vi "MARATHON_CAPACITY TEST.vi"() -> ()   [LabVIEW 2017]
uses:
  <userlib>/LV-Link3/PolySubVIs/DtOLTimingSetInput.vi
  <userlib>/LV-Link3/PolySubVIs/DtOLReadMultiple2D.vi
panel:
  in  "Limit Cell Voltage":dbl[](array[numeric]) format="%_4g"
  out "x+y 2":dbl[](array[numeric])
  out "x+y":dbl[](array[knob]) scale=0.0..32.0
  out "Time 20":dbl format="%<%H:%M:%S>t"
  out "Time 19":dbl format="%<%H:%M:%S>t"
  out "Time 18":dbl format="%<%H:%M:%S>t"
  out "Time 17":dbl format="%<%H:%M:%S>t"
  out "Time 16":dbl format="%<%H:%M:%S>t"
  out "Time 15":dbl format="%<%H:%M:%S>t"
  out "Time 14":dbl format="%<%H:%M:%S>t"
  out "Time 13":dbl format="%<%H:%M:%S>t"
  out "Time 12":dbl format="%<%H:%M:%S>t"
  out "Time 11":dbl format="%<%H:%M:%S>t"
  out "Time 10":dbl format="%<%H:%M:%S>t"
  out "Time 9":dbl format="%<%H:%M:%S>t"
  out "Time 8":dbl format="%<%H:%M:%S>t"
  out "Time 7":dbl format="%<%H:%M:%S>t"
  out "Time 6":dbl format="%<%H:%M:%S>t"
  out "Time 5":dbl format="%<%H:%M:%S>t"
  out "Time 4":dbl format="%<%H:%M:%S>t"
  out "Time 3":dbl format="%<%H:%M:%S>t"
  out "Time 2":dbl format="%<%H:%M:%S>t"
  out "Time 1":dbl format="%<%H:%M:%S>t"
  out "CELL #19":bool[](array[boolean])
  out "CELL #20":bool[](array[boolean])
  out "CELL #18":bool[](array[boolean])
  out "CELL #17":bool[](array[boolean])
  out "CELL #16":bool[](array[boolean])
  out "CELL #15":bool[](array[boolean])
  out "CELL #14":bool[](array[boolean])
  out "CELL #13":bool[](array[boolean])
  out "CELL #12":bool[](array[boolean])
  out "CELL #11":bool[](array[boolean])
  out "CELL #10":bool[](array[boolean])
  out "CELL #9":bool[](array[boolean])
  out "CELL #8":bool[](array[boolean])
  out "CELL #7":bool[](array[boolean])
  out "CELL #6":bool[](array[boolean])
  out "CELL #5":bool[](array[boolean])
  out "CELL #4":bool[](array[boolean])
  out "CELL #3":bool[](array[boolean])
  out "CELL #2":bool[](array[boolean])
  out "CELL #1":bool[](array[boolean])
  out "VOLT # 20":dbl[](array[numeric])
  out "VOLT # 19":dbl[](array[numeric])
  out "VOLT # 18":dbl[](array[numeric])
  out "VOLT # 17":dbl[](array[numeric])
  out "VOLT # 16":dbl[](array[numeric])
  out "VOLT # 15":dbl[](array[numeric])
  out "VOLT # 14":dbl[](array[numeric])
  out "VOLT # 13":dbl[](array[numeric])
  out "VOLT # 12":dbl[](array[numeric])
  out "VOLT # 11":dbl[](array[numeric])
  out "VOLT # 10":dbl[](array[numeric])
  out "VOLT # 9":dbl[](array[numeric])
  out "VOLT # 8":dbl[](array[numeric])
  out "VOLT # 7":dbl[](array[numeric])
  out "VOLT # 6":dbl[](array[numeric])
  out "VOLT # 5":dbl[](array[numeric])
  out "VOLT # 4":dbl[](array[numeric])
  out "VOLT # 3":dbl[](array[numeric])
  out "VOLT # 2":dbl[](array[numeric])
  out "VOLT # 1":dbl[](array[numeric])
  in  "POWER":bool caption="START"
  in  "stop":bool
  # "FLUKE"
  # "179 Multimeter"
  # "28.56789 VOLTS"
  # "SuperMasterCharger"
  # "Time"
  # "Current"
  # "Hold"
  # "Range"
  # "ON"
  # "04:56"
  # "000.7"
  # "R"
  # "20 CELLS"
  # "mV"
  # "Voltage"
  # "D"
  # "V--"
  # "STATUS"
  # "CAP TEST"
  # "A--"
  # "OFF"
  # "Jfm"
  # "1"
  # "Run"
  # "2"
  # "3"
  # "M"
  # "T"
  # "4"
  # "6"
  # "B"
  # "ST"
  # "5"
  # "CU"
  # "SAFT"
  # "8"
  # "OPT"
  # "V"
  # "RST"
  # "7"
  # "9"
  # "Vie"
  # "FN"
  # "ENT"
  # "0"
  # "C"
  # "P"
  # "POWER"
  # "Harness"
  # "WATER"
  # "ACID"
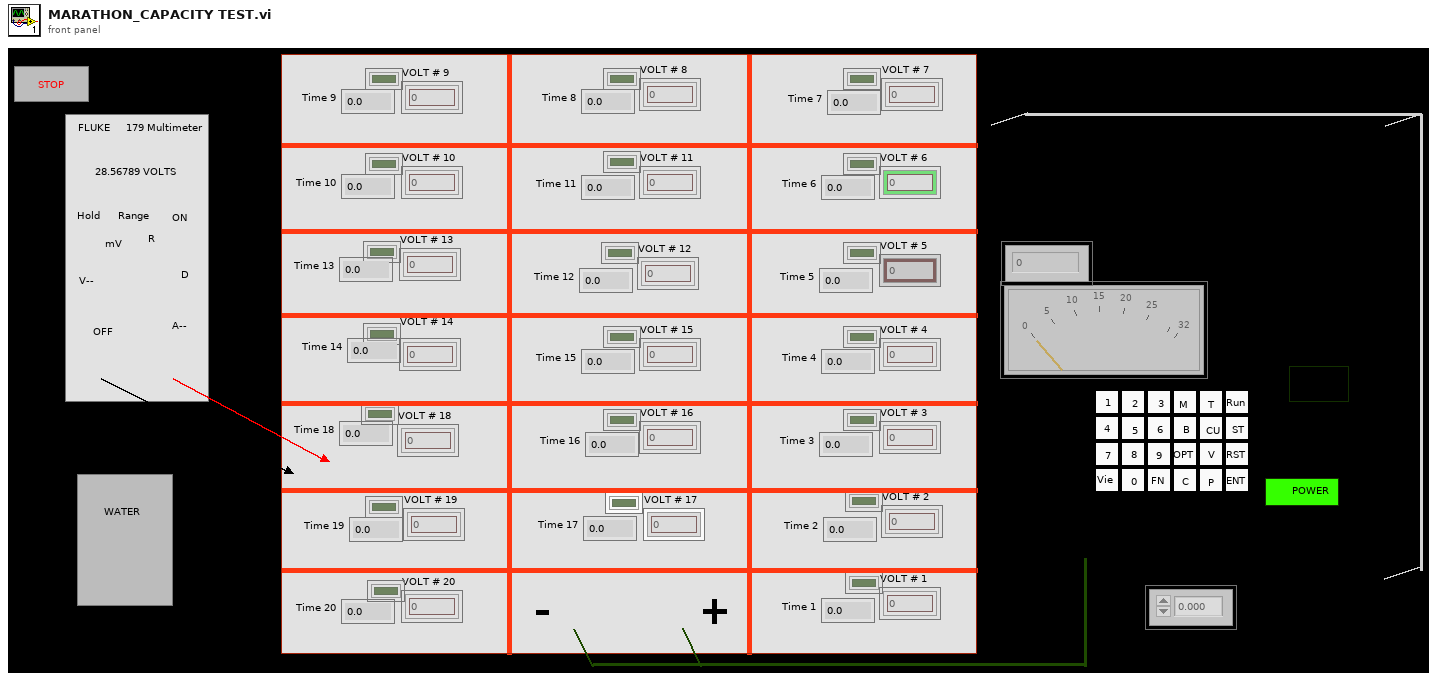
[diagram p1: front panel]
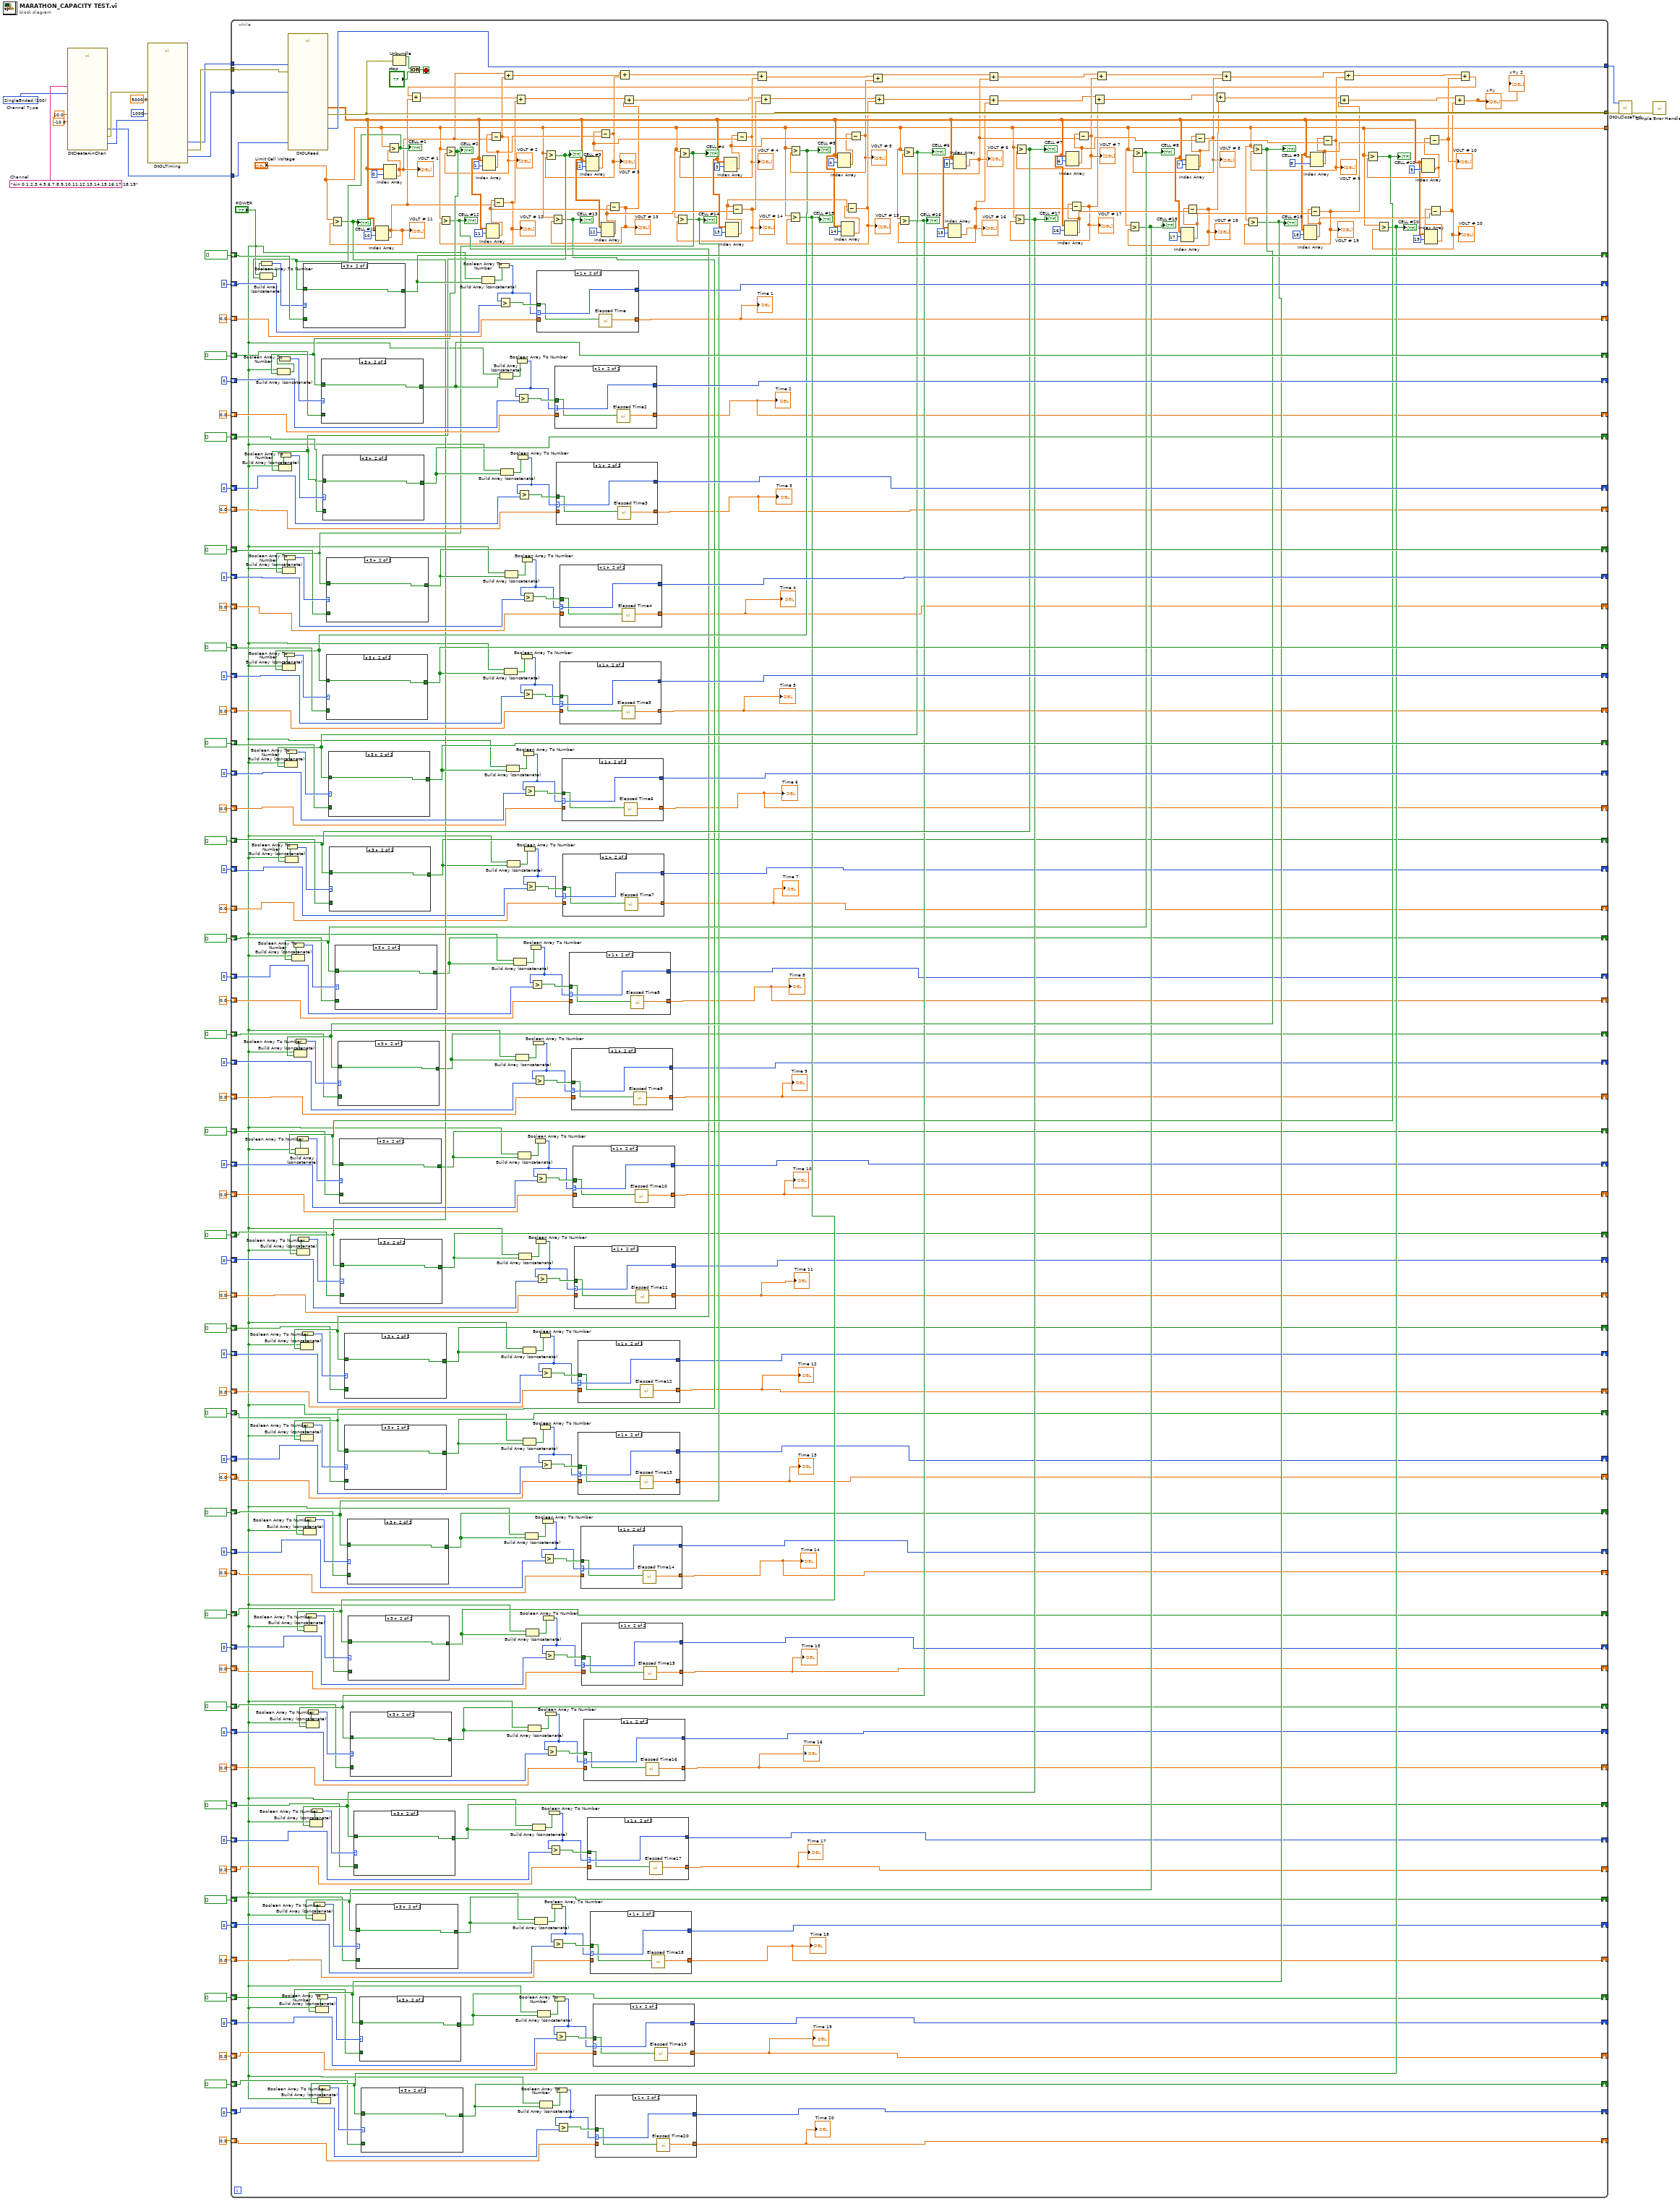
[diagram p0: block diagram]
diagram:
  w75 = 100 items=["Differential"=101, "SingleEnded"=100]  # Channel Type
  w72 = "Ain 0,1,2,3,4,5,6,7,8,9,10,11,12,13,14,15,16,17,18,19"  # Channel
  n1 = call <userlib>:"DtCreateAinChan.vi"("Channel Type"=w75, "Range Min"=-10.0, "Range Max"=10.0, "Channel"=w72) -> ("Task out"=w62:i32, "Actual Number of Channels"=w61:u32, "error out"=w71:errorcluster)  [unwired: 9 in]
  n2 = call-poly <userlib>:"DtOLTiming.vi"("Samples Per Channel"=u32 1000, "error in (no error)"=w71, "Sample Freq (Hz)"=5000.0, "Task in"=w62) -> ("error out"=w68:errorcluster, "Buffer Size"=w67:u32, "Task out"=w66:i32)  [unwired: 4 in, 1 out]
  n3 = while {
    tunnel: w68 -> [w402]
    tunnel: w67 -> [w400]
    tunnel: w66 -> [w401]
    tunnel: [w397] -> w65
    tunnel: [w398] -> w64
    tunnel: w61 -> [w396]
    shift-right: [w255] -> _
    shift-left: bool[] [] -> [w354]
    shift-right: [w214] -> _
    shift-left: u32 0 -> [w353]
    shift-right: [w99] -> _
    shift-left: 0.0 ("Elapsed Time (s)") -> [w352]
    shift-right: [w254] -> _
    shift-left: bool[] [] -> [w253]
    shift-right: [w251] -> _
    shift-left: u32 0 -> [w250]
    shift-right: [w94] -> _
    shift-left: 0.0 ("Elapsed Time (s)") -> [w249]
    shift-right: [w248] -> _
    shift-left: bool[] [] -> [w247]
    shift-right: [w246] -> _
    shift-left: u32 0 -> [w245]
    shift-right: [w93] -> _
    shift-left: 0.0 ("Elapsed Time (s)") -> [w244]
    shift-right: [w243] -> _
    shift-left: bool[] [] -> [w242]
    shift-right: [w241] -> _
    shift-left: u32 0 -> [w240]
    shift-right: [w92] -> _
    shift-left: 0.0 ("Elapsed Time (s)") -> [w239]
    shift-right: [w238] -> _
    shift-left: bool[] [] -> [w236]
    shift-right: [w237] -> _
    shift-left: u32 0 -> [w235]
    shift-right: [w91] -> _
    shift-left: 0.0 ("Elapsed Time (s)") -> [w234]
    shift-right: [w233] -> _
    shift-left: bool[] [] -> [w232]
    shift-right: [w231] -> _
    shift-left: u32 0 -> [w230]
    shift-right: [w90] -> _
    shift-left: 0.0 ("Elapsed Time (s)") -> [w229]
    shift-right: [w206] -> _
    shift-left: bool[] [] -> [w205]
    shift-right: [w204] -> _
    shift-left: u32 0 -> [w203]
    shift-right: [w89] -> _
    shift-left: 0.0 ("Elapsed Time (s)") -> [w202]
    shift-right: [w201] -> _
    shift-left: bool[] [] -> [w175]
    shift-right: [w200] -> _
    shift-left: u32 0 -> [w174]
    shift-right: [w88] -> _
    shift-left: 0.0 ("Elapsed Time (s)") -> [w173]
    shift-right: [w199] -> _
    shift-left: bool[] [] -> [w172]
    shift-right: [w198] -> _
    shift-left: u32 0 -> [w171]
    shift-right: [w87] -> _
    shift-left: 0.0 ("Elapsed Time (s)") -> [w170]
    shift-right: [w197] -> _
    shift-left: bool[] [] -> [w169]
    shift-right: [w196] -> _
    shift-left: u32 0 -> [w168]
    shift-right: [w86] -> _
    shift-left: 0.0 ("Elapsed Time (s)") -> [w167]
    shift-right: [w195] -> _
    shift-left: bool[] [] -> [w166]
    shift-right: [w194] -> _
    shift-left: u32 0 -> [w165]
    shift-right: [w85] -> _
    shift-left: 0.0 ("Elapsed Time (s)") -> [w164]
    shift-right: [w193] -> _
    shift-left: bool[] [] -> [w163]
    shift-right: [w192] -> _
    shift-left: u32 0 -> [w162]
    shift-right: [w84] -> _
    shift-left: 0.0 ("Elapsed Time (s)") -> [w161]
    shift-right: [w191] -> _
    shift-left: bool[] [] -> [w160]
    shift-right: [w190] -> _
    shift-left: u32 0 -> [w159]
    shift-right: [w83] -> _
    shift-left: 0.0 ("Elapsed Time (s)") -> [w158]
    shift-right: [w189] -> _
    shift-left: bool[] [] -> [w157]
    shift-right: [w188] -> _
    shift-left: u32 0 -> [w156]
    shift-right: [w82] -> _
    shift-left: 0.0 ("Elapsed Time (s)") -> [w155]
    shift-right: [w187] -> _
    shift-left: bool[] [] -> [w154]
    shift-right: [w186] -> _
    shift-left: u32 0 -> [w153]
    shift-right: [w81] -> _
    shift-left: 0.0 ("Elapsed Time (s)") -> [w152]
    shift-right: [w185] -> _
    shift-left: bool[] [] -> [w151]
    shift-right: [w184] -> _
    shift-left: u32 0 -> [w150]
    shift-right: [w80] -> _
    shift-left: 0.0 ("Elapsed Time (s)") -> [w149]
    shift-right: [w183] -> _
    shift-left: bool[] [] -> [w148]
    shift-right: [w182] -> _
    shift-left: u32 0 -> [w147]
    shift-right: [w79] -> _
    shift-left: 0.0 ("Elapsed Time (s)") -> [w146]
    shift-right: [w181] -> _
    shift-left: bool[] [] -> [w145]
    shift-right: [w180] -> _
    shift-left: u32 0 -> [w144]
    shift-right: [w78] -> _
    shift-left: 0.0 ("Elapsed Time (s)") -> [w143]
    shift-right: [w179] -> _
    shift-left: bool[] [] -> [w142]
    shift-right: [w178] -> _
    shift-left: u32 0 -> [w141]
    shift-right: [w77] -> _
    shift-left: 0.0 ("Elapsed Time (s)") -> [w140]
    shift-right: [w177] -> _
    shift-left: bool[] [] -> [w139]
    shift-right: [w176] -> _
    shift-left: u32 0 -> [w138]
    shift-right: [w76] -> _
    shift-left: 0.0 ("Elapsed Time (s)") -> [w137]
    tunnel: ["Limit Cell Voltage"] -> _
    stop <- w374 stop-if-true
    n4 = call-poly <userlib>:"DtOLRead.vi"("Number Chan to Read"=w396, "Buffer size"=w400, "error in (no error)"=w402, "Task in"=w401) -> ("error out"=w397:errorcluster, "2D Data out"=w373:dbl[][], "Task out"=w398:i32)  [unwired: 3 in, 2 out]
    n5 = Index Array(array=w373, index (row)=10) -> (element=w97:dbl[])  [unwired: 1 in]
    "VOLT # 11" <- w97
    n6 = Greater?(x="Limit Cell Voltage", y=w97) -> (0:w217:bool[])
    "CELL #11" <- w217
    n7 = Build Array (concatenate)("POWER", w217) -> (w302:bool[])
    n8 = Boolean Array To Number(Boolean array=w302) -> (number=w301:u32)
    n9 = case shown="3" w301 {
      tunnel: w217 -> [_ w472]
      tunnel: [w471 w472] -> w195
      tunnel: w166 -> [w471 _]
      frame 0, Default {
      }
      frame 3 {
      }
    }
    n10 = Index Array(array=w373, index (row)=0) -> (element=w135:dbl[])  [unwired: 1 in]
    "VOLT # 1" <- w135
    n11 = Greater?(x="Limit Cell Voltage", y=w135) -> (0:w228:bool[])
    "CELL #1" <- w228
    n12 = Build Array (concatenate)("POWER", w228) -> (w351:bool[])
    n13 = Boolean Array To Number(Boolean array=w351) -> (number=w350:u32)
    n14 = case shown="3" w350 {
      tunnel: w228 -> [_ w542]
      tunnel: [w541 w542] -> w255
      tunnel: w354 -> [w541 _]
      frame 0, Default {
      }
      frame 3 {
      }
    }
    n15 = Unbundle "Unbundle"(w397) -> ("status"=w399:bool)  [unwired: 2 out]
    n16 = Or(x=w399, y="stop") -> (x .or. y?=w374:bool)
    n17 = Build Array (concatenate)("POWER", w255) -> (w356:bool[])
    n18 = Index Array(array=w373, index (row)=1) -> (element=w372:dbl[])  [unwired: 1 in]
    n19 = Index Array(array=w373, index (row)=11) -> (element=w364:dbl[])  [unwired: 1 in]
    n20 = Subtract(x=w372, y=w135) -> (x-y=w134:dbl[])
    "VOLT # 2" <- w134
    n21 = Greater?(x="Limit Cell Voltage", y=w134) -> (0:w227:bool[])
    "CELL #2" <- w227
    n22 = Build Array (concatenate)("POWER", w227) -> (w252:bool[])
    n23 = Boolean Array To Number(Boolean array=w252) -> (number=w346:u32)
    n24 = case shown="3" w346 {
      tunnel: w227 -> [_ w535]
      tunnel: [w534 w535] -> w254
      tunnel: w253 -> [w534 _]
      frame 0, Default {
      }
      frame 3 {
      }
    }
    n25 = Subtract(x=w364, y=w97) -> (x-y=w116:dbl[])
    "VOLT # 12" <- w116
    n26 = Greater?(x="Limit Cell Voltage", y=w116) -> (0:w216:bool[])
    "CELL #12" <- w216
    n27 = Build Array (concatenate)("POWER", w216) -> (w297:bool[])
    n28 = Boolean Array To Number(Boolean array=w297) -> (number=w296:u32)
    n29 = case shown="3" w296 {
      tunnel: w216 -> [_ w465]
      tunnel: [w464 w465] -> w193
      tunnel: w163 -> [w464 _]
      frame 0, Default {
      }
      frame 3 {
      }
    }
    n30 = Boolean Array To Number(Boolean array=w356) -> (number=w355:u32)
    n31 = Greater?(x=w355, y=w353) -> (0:w357:bool)
    n32 = Build Array (concatenate)("POWER", w254) -> (w348:bool[])
    n33 = Add(x=w135, y=w134) -> (x+y=w133:dbl[])
    n34 = Boolean Array To Number(Boolean array=w348) -> (number=w347:u32)
    n35 = Greater?(x=w347, y=w250) -> (0:w349:bool)
    n36 = Build Array (concatenate)("POWER", w195) -> (w304:bool[])
    n37 = Build Array (concatenate)("POWER", w193) -> (w299:bool[])
    n38 = Boolean Array To Number(Boolean array=w304) -> (number=w303:u32)
    n39 = Greater?(x=w303, y=w165) -> (0:w305:bool)
    n40 = case shown="1" w355 {
      selector: w355 -> [w537 w539]
      tunnel: [w536 w540] -> w99
      tunnel: w352 -> [w536 _]
      tunnel: [w537 w539] -> w214
      tunnel: w357 -> [_ w538]
      frame 0, Default {
      }
      frame 1 {
        n41 = call "Elapsed Time"("Reset"=w538) -> ("Elapsed Time (s)"=w540:dbl)  [unwired: 11 in, 7 out]
      }
    }
    "Time 1" <- w99
    n42 = Boolean Array To Number(Boolean array=w299) -> (number=w298:u32)
    n43 = Greater?(x=w298, y=w162) -> (0:w300:bool)
    n44 = case shown="1" w347 {
      selector: w347 -> [w530 w532]
      tunnel: [w529 w533] -> w94
      tunnel: w249 -> [w529 _]
      tunnel: [w530 w532] -> w251
      tunnel: w349 -> [_ w531]
      frame 0, Default {
      }
      frame 1 {
        n45 = call "Elapsed Time2"("Reset"=w531) -> ("Elapsed Time (s)"=w533:dbl)  [unwired: 11 in, 7 out]
      }
    }
    "Time 2" <- w94
    n46 = case shown="1" w303 {
      selector: w303 -> [w467 w469]
      tunnel: [w466 w470] -> w85
      tunnel: w164 -> [w466 _]
      tunnel: [w467 w469] -> w194
      tunnel: w305 -> [_ w468]
      frame 0, Default {
      }
      frame 1 {
        n47 = call "Elapsed Time11"("Reset"=w468) -> ("Elapsed Time (s)"=w470:dbl)  [unwired: 11 in, 7 out]
      }
    }
    "Time 11" <- w85
    n48 = case shown="1" w298 {
      selector: w298 -> [w460 w462]
      tunnel: [w459 w463] -> w84
      tunnel: w161 -> [w459 _]
      tunnel: [w460 w462] -> w192
      tunnel: w300 -> [_ w461]
      frame 0, Default {
      }
      frame 1 {
        n49 = call "Elapsed Time12"("Reset"=w461) -> ("Elapsed Time (s)"=w463:dbl)  [unwired: 11 in, 7 out]
      }
    }
    "Time 12" <- w84
    n50 = Index Array(array=w373, index (row)=2) -> (element=w371:dbl[])  [unwired: 1 in]
    n51 = Subtract(x=w371, y=w372) -> (x-y=w132:dbl[])
    "VOLT # 3" <- w132
    n52 = Greater?(x="Limit Cell Voltage", y=w132) -> (0:w226:bool[])
    "CELL #3" <- w226
    n53 = Build Array (concatenate)("POWER", w226) -> (w342:bool[])
    n54 = Boolean Array To Number(Boolean array=w342) -> (number=w341:u32)
    n55 = case shown="3" w341 {
      tunnel: w226 -> [_ w528]
      tunnel: [w527 w528] -> w248
      tunnel: w247 -> [w527 _]
      frame 0, Default {
      }
      frame 3 {
      }
    }
    n56 = Build Array (concatenate)("POWER", w248) -> (w344:bool[])
    n57 = Boolean Array To Number(Boolean array=w344) -> (number=w343:u32)
    n58 = Greater?(x=w343, y=w245) -> (0:w345:bool)
    n59 = case shown="1" w343 {
      selector: w343 -> [w523 w525]
      tunnel: [w522 w526] -> w93
      tunnel: w244 -> [w522 _]
      tunnel: [w523 w525] -> w246
      tunnel: w345 -> [_ w524]
      frame 0, Default {
      }
      frame 1 {
        n60 = call "Elapsed Time3"("Reset"=w524) -> ("Elapsed Time (s)"=w526:dbl)  [unwired: 11 in, 7 out]
      }
    }
    "Time 3" <- w93
    n61 = Index Array(array=w373, index (row)=12) -> (element=w225:dbl[])  [unwired: 1 in]
    n62 = Subtract(x=w225, y=w364) -> (x-y=w114:dbl[])
    "VOLT # 13" <- w114
    n63 = Greater?(x="Limit Cell Voltage", y=w114) -> (0:w215:bool[])
    "CELL #13" <- w215
    n64 = Build Array (concatenate)("POWER", w215) -> (w292:bool[])
    n65 = Boolean Array To Number(Boolean array=w292) -> (number=w291:u32)
    n66 = case shown="3" w291 {
      tunnel: w215 -> [_ w458]
      tunnel: [w457 w458] -> w191
      tunnel: w160 -> [w457 _]
      frame 0, Default {
      }
      frame 3 {
      }
    }
    n67 = Build Array (concatenate)("POWER", w191) -> (w294:bool[])
    n68 = Boolean Array To Number(Boolean array=w294) -> (number=w293:u32)
    n69 = Greater?(x=w293, y=w159) -> (0:w295:bool)
    n70 = case shown="1" w293 {
      selector: w293 -> [w453 w455]
      tunnel: [w452 w456] -> w83
      tunnel: w158 -> [w452 _]
      tunnel: [w453 w455] -> w190
      tunnel: w295 -> [_ w454]
      frame 0, Default {
      }
      frame 1 {
        n71 = call "Elapsed Time13"("Reset"=w454) -> ("Elapsed Time (s)"=w456:dbl)  [unwired: 11 in, 7 out]
      }
    }
    "Time 13" <- w83
    n72 = Add(x=w133, y=w132) -> (x+y=w131:dbl[])
    n73 = Index Array(array=w373, index (row)=3) -> (element=w370:dbl[])  [unwired: 1 in]
    n74 = Index Array(array=w373, index (row)=13) -> (element=w363:dbl[])  [unwired: 1 in]
    n75 = Subtract(x=w363, y=w225) -> (x-y=w112:dbl[])
    "VOLT # 14" <- w112
    n76 = Greater?(x="Limit Cell Voltage", y=w112) -> (0:w213:bool[])
    "CELL #14" <- w213
    n77 = Build Array (concatenate)("POWER", w213) -> (w287:bool[])
    n78 = Boolean Array To Number(Boolean array=w287) -> (number=w286:u32)
    n79 = case shown="3" w286 {
      tunnel: w213 -> [_ w451]
      tunnel: [w450 w451] -> w189
      tunnel: w157 -> [w450 _]
      frame 0, Default {
      }
      frame 3 {
      }
    }
    n80 = Build Array (concatenate)("POWER", w189) -> (w289:bool[])
    n81 = Boolean Array To Number(Boolean array=w289) -> (number=w288:u32)
    n82 = Greater?(x=w288, y=w156) -> (0:w290:bool)
    n83 = case shown="1" w288 {
      selector: w288 -> [w446 w448]
      tunnel: [w445 w449] -> w82
      tunnel: w155 -> [w445 _]
      tunnel: [w446 w448] -> w188
      tunnel: w290 -> [_ w447]
      frame 0, Default {
      }
      frame 1 {
        n84 = call "Elapsed Time14"("Reset"=w447) -> ("Elapsed Time (s)"=w449:dbl)  [unwired: 11 in, 7 out]
      }
    }
    "Time 14" <- w82
    n85 = Subtract(x=w370, y=w371) -> (x-y=w130:dbl[])
    "VOLT # 4" <- w130
    n86 = Greater?(x="Limit Cell Voltage", y=w130) -> (0:w224:bool[])
    "CELL #4" <- w224
    n87 = Build Array (concatenate)("POWER", w224) -> (w337:bool[])
    n88 = Boolean Array To Number(Boolean array=w337) -> (number=w336:u32)
    n89 = case shown="3" w336 {
      tunnel: w224 -> [_ w521]
      tunnel: [w520 w521] -> w243
      tunnel: w242 -> [w520 _]
      frame 0, Default {
      }
      frame 3 {
      }
    }
    n90 = Build Array (concatenate)("POWER", w243) -> (w339:bool[])
    n91 = Boolean Array To Number(Boolean array=w339) -> (number=w338:u32)
    n92 = Greater?(x=w338, y=w240) -> (0:w340:bool)
    n93 = case shown="1" w338 {
      selector: w338 -> [w516 w518]
      tunnel: [w515 w519] -> w92
      tunnel: w239 -> [w515 _]
      tunnel: [w516 w518] -> w241
      tunnel: w340 -> [_ w517]
      frame 0, Default {
      }
      frame 1 {
        n94 = call "Elapsed Time4"("Reset"=w517) -> ("Elapsed Time (s)"=w519:dbl)  [unwired: 11 in, 7 out]
      }
    }
    "Time 4" <- w92
    n95 = Add(x=w131, y=w130) -> (x+y=w129:dbl[])
    n96 = Index Array(array=w373, index (row)=4) -> (element=w369:dbl[])  [unwired: 1 in]
    n97 = Index Array(array=w373, index (row)=14) -> (element=w362:dbl[])  [unwired: 1 in]
    n98 = Subtract(x=w362, y=w363) -> (x-y=w110:dbl[])
    "VOLT # 15" <- w110
    n99 = Greater?(x="Limit Cell Voltage", y=w110) -> (0:w212:bool[])
    "CELL #15" <- w212
    n100 = Build Array (concatenate)("POWER", w212) -> (w282:bool[])
    n101 = Boolean Array To Number(Boolean array=w282) -> (number=w281:u32)
    n102 = case shown="3" w281 {
      tunnel: w212 -> [_ w444]
      tunnel: [w443 w444] -> w187
      tunnel: w154 -> [w443 _]
      frame 0, Default {
      }
      frame 3 {
      }
    }
    n103 = Build Array (concatenate)("POWER", w187) -> (w284:bool[])
    n104 = Boolean Array To Number(Boolean array=w284) -> (number=w283:u32)
    n105 = Greater?(x=w283, y=w153) -> (0:w285:bool)
    n106 = case shown="1" w283 {
      selector: w283 -> [w439 w441]
      tunnel: [w438 w442] -> w81
      tunnel: w152 -> [w438 _]
      tunnel: [w439 w441] -> w186
      tunnel: w285 -> [_ w440]
      frame 0, Default {
      }
      frame 1 {
        n107 = call "Elapsed Time15"("Reset"=w440) -> ("Elapsed Time (s)"=w442:dbl)  [unwired: 11 in, 7 out]
      }
    }
    "Time 15" <- w81
    n108 = Subtract(x=w369, y=w370) -> (x-y=w128:dbl[])
    "VOLT # 5" <- w128
    n109 = Greater?(x="Limit Cell Voltage", y=w128) -> (0:w223:bool[])
    "CELL #5" <- w223
    n110 = Build Array (concatenate)("POWER", w223) -> (w332:bool[])
    n111 = Boolean Array To Number(Boolean array=w332) -> (number=w331:u32)
    n112 = case shown="3" w331 {
      tunnel: w223 -> [_ w514]
      tunnel: [w513 w514] -> w238
      tunnel: w236 -> [w513 _]
      frame 0, Default {
      }
      frame 3 {
      }
    }
    n113 = Build Array (concatenate)("POWER", w238) -> (w334:bool[])
    n114 = Boolean Array To Number(Boolean array=w334) -> (number=w333:u32)
    n115 = Greater?(x=w333, y=w235) -> (0:w335:bool)
    n116 = case shown="1" w333 {
      selector: w333 -> [w509 w511]
      tunnel: [w508 w512] -> w91
      tunnel: w234 -> [w508 _]
      tunnel: [w509 w511] -> w237
      tunnel: w335 -> [_ w510]
      frame 0, Default {
      }
      frame 1 {
        n117 = call "Elapsed Time5"("Reset"=w510) -> ("Elapsed Time (s)"=w512:dbl)  [unwired: 11 in, 7 out]
      }
    }
    "Time 5" <- w91
    n118 = Add(x=w129, y=w128) -> (x+y=w127:dbl[])
    n119 = Index Array(array=w373, index (row)=15) -> (element=w96:dbl[])  [unwired: 1 in]
    "VOLT # 16" <- w96
    n120 = Greater?(x="Limit Cell Voltage", y=w96) -> (0:w211:bool[])
    "CELL #16" <- w211
    n121 = Build Array (concatenate)("POWER", w211) -> (w277:bool[])
    n122 = Boolean Array To Number(Boolean array=w277) -> (number=w276:u32)
    n123 = case shown="3" w276 {
      tunnel: w211 -> [_ w437]
      tunnel: [w436 w437] -> w185
      tunnel: w151 -> [w436 _]
      frame 0, Default {
      }
      frame 3 {
      }
    }
    n124 = Build Array (concatenate)("POWER", w185) -> (w279:bool[])
    n125 = Boolean Array To Number(Boolean array=w279) -> (number=w278:u32)
    n126 = Greater?(x=w278, y=w150) -> (0:w280:bool)
    n127 = case shown="1" w278 {
      selector: w278 -> [w432 w434]
      tunnel: [w431 w435] -> w80
      tunnel: w149 -> [w431 _]
      tunnel: [w432 w434] -> w184
      tunnel: w280 -> [_ w433]
      frame 0, Default {
      }
      frame 1 {
        n128 = call "Elapsed Time16"("Reset"=w433) -> ("Elapsed Time (s)"=w435:dbl)  [unwired: 11 in, 7 out]
      }
    }
    "Time 16" <- w80
    n129 = Index Array(array=w373, index (row)=5) -> (element=w98:dbl[])  [unwired: 1 in]
    "VOLT # 6" <- w98
    n130 = Greater?(x="Limit Cell Voltage", y=w98) -> (0:w222:bool[])
    "CELL #6" <- w222
    n131 = Build Array (concatenate)("POWER", w222) -> (w327:bool[])
    n132 = Boolean Array To Number(Boolean array=w327) -> (number=w326:u32)
    n133 = case shown="3" w326 {
      tunnel: w222 -> [_ w507]
      tunnel: [w506 w507] -> w233
      tunnel: w232 -> [w506 _]
      frame 0, Default {
      }
      frame 3 {
      }
    }
    n134 = Build Array (concatenate)("POWER", w233) -> (w329:bool[])
    n135 = Boolean Array To Number(Boolean array=w329) -> (number=w328:u32)
    n136 = Greater?(x=w328, y=w230) -> (0:w330:bool)
    n137 = case shown="1" w328 {
      selector: w328 -> [w502 w504]
      tunnel: [w501 w505] -> w90
      tunnel: w229 -> [w501 _]
      tunnel: [w502 w504] -> w231
      tunnel: w330 -> [_ w503]
      frame 0, Default {
      }
      frame 1 {
        n138 = call "Elapsed Time6"("Reset"=w503) -> ("Elapsed Time (s)"=w505:dbl)  [unwired: 11 in, 7 out]
      }
    }
    "Time 6" <- w90
    n139 = Add(x=w127, y=w98) -> (x+y=w126:dbl[])
    n140 = Index Array(array=w373, index (row)=16) -> (element=w361:dbl[])  [unwired: 1 in]
    n141 = Index Array(array=w373, index (row)=6) -> (element=w368:dbl[])  [unwired: 1 in]
    n142 = Subtract(x=w361, y=w96) -> (x-y=w107:dbl[])
    "VOLT # 17" <- w107
    n143 = Greater?(x="Limit Cell Voltage", y=w107) -> (0:w210:bool[])
    "CELL #17" <- w210
    n144 = Build Array (concatenate)("POWER", w210) -> (w272:bool[])
    n145 = Boolean Array To Number(Boolean array=w272) -> (number=w271:u32)
    n146 = case shown="3" w271 {
      tunnel: w210 -> [_ w430]
      tunnel: [w429 w430] -> w183
      tunnel: w148 -> [w429 _]
      frame 0, Default {
      }
      frame 3 {
      }
    }
    n147 = Build Array (concatenate)("POWER", w183) -> (w274:bool[])
    n148 = Boolean Array To Number(Boolean array=w274) -> (number=w273:u32)
    n149 = Greater?(x=w273, y=w147) -> (0:w275:bool)
    n150 = case shown="1" w273 {
      selector: w273 -> [w425 w427]
      tunnel: [w424 w428] -> w79
      tunnel: w146 -> [w424 _]
      tunnel: [w425 w427] -> w182
      tunnel: w275 -> [_ w426]
      frame 0, Default {
      }
      frame 1 {
        n151 = call "Elapsed Time17"("Reset"=w426) -> ("Elapsed Time (s)"=w428:dbl)  [unwired: 11 in, 7 out]
      }
    }
    "Time 17" <- w79
    n152 = Subtract(x=w368, y=w98) -> (x-y=w125:dbl[])
    "VOLT # 7" <- w125
    n153 = Greater?(x="Limit Cell Voltage", y=w125) -> (0:w221:bool[])
    "CELL #7" <- w221
    n154 = Build Array (concatenate)("POWER", w221) -> (w322:bool[])
    n155 = Boolean Array To Number(Boolean array=w322) -> (number=w321:u32)
    n156 = case shown="3" w321 {
      tunnel: w221 -> [_ w500]
      tunnel: [w499 w500] -> w206
      tunnel: w205 -> [w499 _]
      frame 0, Default {
      }
      frame 3 {
      }
    }
    n157 = Build Array (concatenate)("POWER", w206) -> (w324:bool[])
    n158 = Boolean Array To Number(Boolean array=w324) -> (number=w323:u32)
    n159 = Greater?(x=w323, y=w203) -> (0:w325:bool)
    n160 = case shown="1" w323 {
      selector: w323 -> [w495 w497]
      tunnel: [w494 w498] -> w89
      tunnel: w202 -> [w494 _]
      tunnel: [w495 w497] -> w204
      tunnel: w325 -> [_ w496]
      frame 0, Default {
      }
      frame 1 {
        n161 = call "Elapsed Time7"("Reset"=w496) -> ("Elapsed Time (s)"=w498:dbl)  [unwired: 11 in, 7 out]
      }
    }
    "Time 7" <- w89
    n162 = Add(x=w126, y=w125) -> (x+y=w124:dbl[])
    n163 = Index Array(array=w373, index (row)=17) -> (element=w360:dbl[])  [unwired: 1 in]
    n164 = Index Array(array=w373, index (row)=7) -> (element=w367:dbl[])  [unwired: 1 in]
    n165 = Subtract(x=w360, y=w361) -> (x-y=w105:dbl[])
    "VOLT # 18" <- w105
    n166 = Greater?(x="Limit Cell Voltage", y=w105) -> (0:w209:bool[])
    "CELL #18" <- w209
    n167 = Build Array (concatenate)("POWER", w209) -> (w267:bool[])
    n168 = Boolean Array To Number(Boolean array=w267) -> (number=w266:u32)
    n169 = case shown="3" w266 {
      tunnel: w209 -> [_ w423]
      tunnel: [w422 w423] -> w181
      tunnel: w145 -> [w422 _]
      frame 0, Default {
      }
      frame 3 {
      }
    }
    n170 = Build Array (concatenate)("POWER", w181) -> (w269:bool[])
    n171 = Boolean Array To Number(Boolean array=w269) -> (number=w268:u32)
    n172 = Greater?(x=w268, y=w144) -> (0:w270:bool)
    n173 = case shown="1" w268 {
      selector: w268 -> [w418 w420]
      tunnel: [w417 w421] -> w78
      tunnel: w143 -> [w417 _]
      tunnel: [w418 w420] -> w180
      tunnel: w270 -> [_ w419]
      frame 0, Default {
      }
      frame 1 {
        n174 = call "Elapsed Time18"("Reset"=w419) -> ("Elapsed Time (s)"=w421:dbl)  [unwired: 11 in, 7 out]
      }
    }
    "Time 18" <- w78
    n175 = Subtract(x=w367, y=w368) -> (x-y=w123:dbl[])
    "VOLT # 8" <- w123
    n176 = Greater?(x="Limit Cell Voltage", y=w123) -> (0:w220:bool[])
    "CELL #8" <- w220
    n177 = Build Array (concatenate)("POWER", w220) -> (w317:bool[])
    n178 = Boolean Array To Number(Boolean array=w317) -> (number=w316:u32)
    n179 = case shown="3" w316 {
      tunnel: w220 -> [_ w493]
      tunnel: [w492 w493] -> w201
      tunnel: w175 -> [w492 _]
      frame 0, Default {
      }
      frame 3 {
      }
    }
    n180 = Build Array (concatenate)("POWER", w201) -> (w319:bool[])
    n181 = Boolean Array To Number(Boolean array=w319) -> (number=w318:u32)
    n182 = Greater?(x=w318, y=w174) -> (0:w320:bool)
    n183 = case shown="1" w318 {
      selector: w318 -> [w488 w490]
      tunnel: [w487 w491] -> w88
      tunnel: w173 -> [w487 _]
      tunnel: [w488 w490] -> w200
      tunnel: w320 -> [_ w489]
      frame 0, Default {
      }
      frame 1 {
        n184 = call "Elapsed Time8"("Reset"=w489) -> ("Elapsed Time (s)"=w491:dbl)  [unwired: 11 in, 7 out]
      }
    }
    "Time 8" <- w88
    n185 = Add(x=w124, y=w123) -> (x+y=w122:dbl[])
    n186 = Index Array(array=w373, index (row)=18) -> (element=w359:dbl[])  [unwired: 1 in]
    n187 = Subtract(x=w359, y=w360) -> (x-y=w103:dbl[])
    "VOLT # 19" <- w103
    n188 = Greater?(x="Limit Cell Voltage", y=w103) -> (0:w208:bool[])
    "CELL #19" <- w208
    n189 = Build Array (concatenate)("POWER", w208) -> (w262:bool[])
    n190 = Boolean Array To Number(Boolean array=w262) -> (number=w261:u32)
    n191 = case shown="3" w261 {
      tunnel: w208 -> [_ w416]
      tunnel: [w415 w416] -> w179
      tunnel: w142 -> [w415 _]
      frame 0, Default {
      }
      frame 3 {
      }
    }
    n192 = Build Array (concatenate)("POWER", w179) -> (w264:bool[])
    n193 = Boolean Array To Number(Boolean array=w264) -> (number=w263:u32)
    n194 = Greater?(x=w263, y=w141) -> (0:w265:bool)
    n195 = case shown="1" w263 {
      selector: w263 -> [w411 w413]
      tunnel: [w410 w414] -> w77
      tunnel: w140 -> [w410 _]
      tunnel: [w411 w413] -> w178
      tunnel: w265 -> [_ w412]
      frame 0, Default {
      }
      frame 1 {
        n196 = call "Elapsed Time19"("Reset"=w412) -> ("Elapsed Time (s)"=w414:dbl)  [unwired: 11 in, 7 out]
      }
    }
    "Time 19" <- w77
    n197 = Index Array(array=w373, index (row)=8) -> (element=w366:dbl[])  [unwired: 1 in]
    n198 = Subtract(x=w366, y=w367) -> (x-y=w121:dbl[])
    "VOLT # 9" <- w121
    n199 = Greater?(x="Limit Cell Voltage", y=w121) -> (0:w219:bool[])
    "CELL #9" <- w219
    n200 = Build Array (concatenate)("POWER", w219) -> (w312:bool[])
    n201 = Boolean Array To Number(Boolean array=w312) -> (number=w311:u32)
    n202 = case shown="3" w311 {
      tunnel: w219 -> [_ w486]
      tunnel: [w485 w486] -> w199
      tunnel: w172 -> [w485 _]
      frame 0, Default {
      }
      frame 3 {
      }
    }
    n203 = Build Array (concatenate)("POWER", w199) -> (w314:bool[])
    n204 = Boolean Array To Number(Boolean array=w314) -> (number=w313:u32)
    n205 = Greater?(x=w313, y=w171) -> (0:w315:bool)
    n206 = case shown="1" w313 {
      selector: w313 -> [w481 w483]
      tunnel: [w480 w484] -> w87
      tunnel: w170 -> [w480 _]
      tunnel: [w481 w483] -> w198
      tunnel: w315 -> [_ w482]
      frame 0, Default {
      }
      frame 1 {
        n207 = call "Elapsed Time9"("Reset"=w482) -> ("Elapsed Time (s)"=w484:dbl)  [unwired: 11 in, 7 out]
      }
    }
    "Time 9" <- w87
    n208 = Add(x=w122, y=w121) -> (x+y=w120:dbl[])
    n209 = Index Array(array=w373, index (row)=9) -> (element=w365:dbl[])  [unwired: 1 in]
    n210 = Greater?(x="Limit Cell Voltage", y=w365) -> (0:w218:bool[])
    "CELL #10" <- w218
    n211 = Build Array (concatenate)("POWER", w218) -> (w307:bool[])
    n212 = Boolean Array To Number(Boolean array=w307) -> (number=w306:u32)
    n213 = case shown="3" w306 {
      tunnel: w218 -> [_ w479]
      tunnel: [w478 w479] -> w197
      tunnel: w169 -> [w478 _]
      frame 0, Default {
      }
      frame 3 {
      }
    }
    n214 = Build Array (concatenate)("POWER", w197) -> (w309:bool[])
    n215 = Boolean Array To Number(Boolean array=w309) -> (number=w308:u32)
    n216 = Greater?(x=w308, y=w168) -> (0:w310:bool)
    n217 = case shown="1" w308 {
      selector: w308 -> [w474 w476]
      tunnel: [w473 w477] -> w86
      tunnel: w167 -> [w473 _]
      tunnel: [w474 w476] -> w196
      tunnel: w310 -> [_ w475]
      frame 0, Default {
      }
      frame 1 {
        n218 = call "Elapsed Time10"("Reset"=w475) -> ("Elapsed Time (s)"=w477:dbl)  [unwired: 11 in, 7 out]
      }
    }
    "Time 10" <- w86
    n219 = Index Array(array=w373, index (row)=19) -> (element=w358:dbl[])  [unwired: 1 in]
    n220 = Subtract(x=w365, y=w366) -> (x-y=w119:dbl[])
    "VOLT # 10" <- w119
    n221 = Subtract(x=w358, y=w359) -> (x-y=w101:dbl[])
    "VOLT # 20" <- w101
    n222 = Greater?(x="Limit Cell Voltage", y=w101) -> (0:w207:bool[])
    "CELL #20" <- w207
    n223 = Build Array (concatenate)("POWER", w207) -> (w257:bool[])
    n224 = Boolean Array To Number(Boolean array=w257) -> (number=w256:u32)
    n225 = case shown="3" w256 {
      tunnel: w207 -> [_ w409]
      tunnel: [w408 w409] -> w177
      tunnel: w139 -> [w408 _]
      frame 0, Default {
      }
      frame 3 {
      }
    }
    n226 = Build Array (concatenate)("POWER", w177) -> (w259:bool[])
    n227 = Boolean Array To Number(Boolean array=w259) -> (number=w258:u32)
    n228 = Greater?(x=w258, y=w138) -> (0:w260:bool)
    n229 = case shown="1" w258 {
      selector: w258 -> [w404 w406]
      tunnel: [w403 w407] -> w76
      tunnel: w137 -> [w403 _]
      tunnel: [w404 w406] -> w176
      tunnel: w260 -> [_ w405]
      frame 0, Default {
      }
      frame 1 {
        n230 = call "Elapsed Time20"("Reset"=w405) -> ("Elapsed Time (s)"=w407:dbl)  [unwired: 11 in, 7 out]
      }
    }
    "Time 20" <- w76
    n231 = Add(x=w120, y=w119) -> (x+y=w118:dbl[])
    n232 = Add(x=w118, y=w97) -> (x+y=w117:dbl[])
    n233 = Add(x=w117, y=w116) -> (x+y=w115:dbl[])
    n234 = Add(x=w115, y=w114) -> (x+y=w113:dbl[])
    n235 = Add(x=w113, y=w112) -> (x+y=w111:dbl[])
    n236 = Add(x=w111, y=w110) -> (x+y=w109:dbl[])
    n237 = Add(x=w109, y=w96) -> (x+y=w108:dbl[])
    n238 = Add(x=w108, y=w107) -> (x+y=w106:dbl[])
    n239 = Add(x=w106, y=w105) -> (x+y=w104:dbl[])
    n240 = Add(x=w104, y=w103) -> (x+y=w102:dbl[])
    n241 = Add(x=w102, y=w101) -> (x+y=→"x+y" →"x+y 2":dbl[])
  }
  n242 = call <userlib>:"DtOLCloseTask.vi"("Error in"=w65, "Task in"=w64) -> ("Error Out"=w63:errorcluster)  [unwired: 9 in]
  n243 = call <vilib>:"Simple Error Handler.vi"("error in (no error)"=w63) -> ()  [unwired: 4 in, 5 out]
